vi "Handle Ready State.vi"(0 "reference in":refnum<class "PM_Group.lvclass">, 11 "error in (no error)":errorcluster) -> (4 "reference out":refnum<class "PM_Group.lvclass">, 15 "error out":errorcluster)   [LabVIEW 2019, in "PM_Group.lvclass"]
uses:
  PM_Group.lvclass
  C:/Users/H4001/Documents/GitHub/H4000/src/Device_class/Device.lvclass
  PM_Group.lvclass/PM_Group.ctl
  Device_class/Device.lvclass/Device.ctl
  FPGA/TypeDef/DI index.ctl
  TypeDef/State PMG.ctl
  FPGA_API_class/FPGA API.lvclass
  Device_class/Device.lvclass
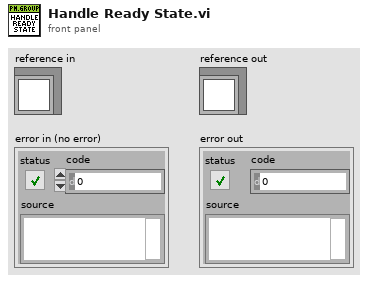
[diagram p1: front panel]
types:
  T1 = typedef "State PMG.ctl" = enum16{"NOT READY", "IDLE", "ACTIVE", "ERROR"}
  T2 = typedef "DI index.ctl" = u8
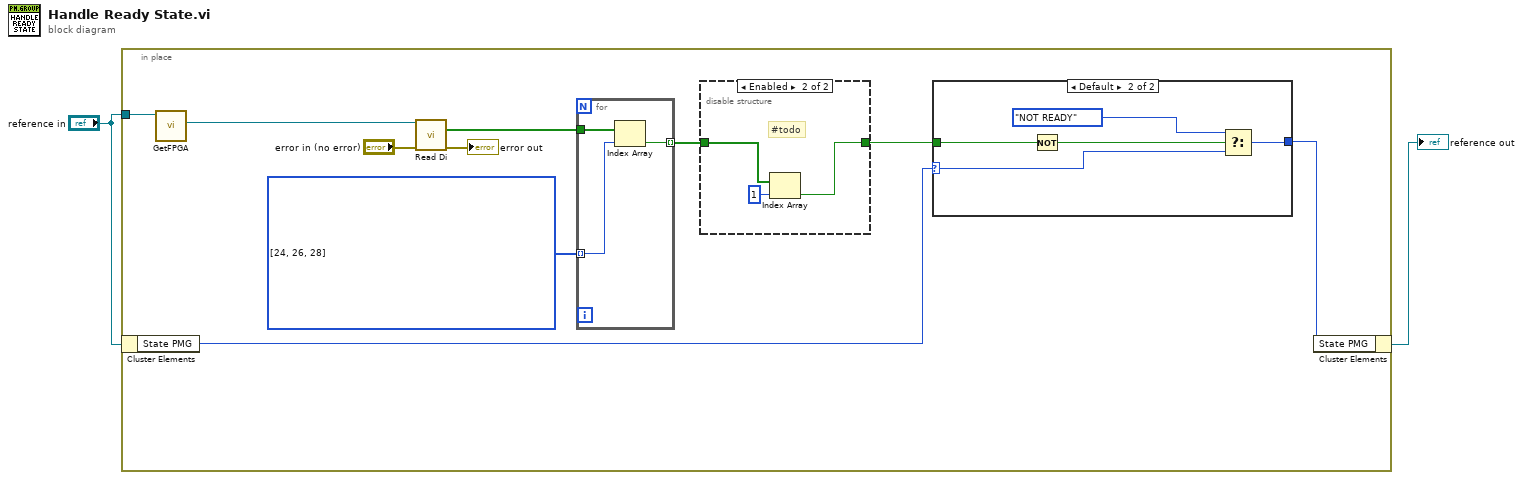
[diagram p0: block diagram]
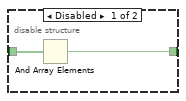
[diagram p2: hidden frame]
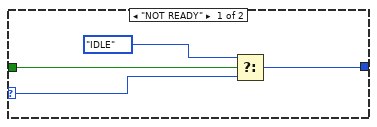
[diagram p3: hidden frame]
diagram:
  n1 = in-place {
    in-place-border: "reference in" -> [w4]
    w11 = T2[] [24, 26, 28] items=["DI 0 [QF1]", "DI 1 [QF2]", "DI 2 [QF3]", "DI 3 [QF4]", "DI 4 [QF5]", "DI 5 [QF6]", "DI 6 [QF7]", "DI 7 [QF8]", "DI 8 [QF9]", "DI 9 [PHASE CONTROL RELAY CONTACTOR [KV1]]", "DI 10 [G1]", "DI 11 [G2]", "DI 12 [RESET BTN [SB1]]", "DI 13 [START BTN [SB2]]", "DI 14 [STOP BTN [SB3]]", "DI 15 [ES BTN [SB4]]", "DI 16 [MANUAL/AUTO MODE SA1]", "DI 17 [[S1]]", "DI 18 [[S2]]", "DI 19 [[S3]]", "DI 20 [[S4]]", "DI 21 [44.1 OPEN]", "DI 22 [44.1 CLOSE]", "DI 23 [CONTACTOR [MK1]]", "DI 24 [AUTOMATIC [QF11]]", "DI 25 [CONTACTOR [MK2]]", "DI 26 [AUTOMATIC [QF12]]", "DI 27 [CONTACTOR [MK3]]", "DI 28 [AUTOMATIC [QF13]]", "DI 29 [44.2 OPEN]", "DI 30 [44.2 CLOSE]"] ("Array")
    n2 = in-place-cluster #1("reference in") -> ("State PMG"=w9:T1)
    n3 = call "GetFPGA.vi"("Device in"=w4) -> ("FPGA API.lvclass"=w3:refnum<class "FPGA API.lvclass">)  [unwired: 10 in]
    n4 = call "Read Di.vi"("FPGA API in"=w3, "error in (no error)"="error in (no error)") -> ("DIs"=w12:bool[], "error out"=→"error out":errorcluster)  [unwired: 11 in, 1 out]
    n5 = for {
      tunnel: w12 -> [w29]
      tunnel: w11 -> [w28] mode=indexing
      tunnel: [w27] -> w10 mode=indexing
      n6 = Index Array(array=w29, index=w28) -> (element=w27:bool)
    }
    n7 = disable-structure shown="Enabled" {
      disable-tunnel: w10 -> [w14 w17]
      disable-tunnel: [w13 w15] -> w8
      frame Disabled {
        n8 = And Array Elements(Boolean array=w14) -> (logical AND=w13:bool)
      }
      frame Enabled {
        # "#todo"
        n9 = Index Array(array=w17, index=1) -> (element=w15:bool)
      }
    }
    n10 = case shown="Default" w9 {
      selector: w9 -> [w20 w25]
      tunnel: w8 -> [w21 w26]
      tunnel: [w18 w23] -> w7
      frame "NOT READY" {
        n11 = Select(t=State_PMG."IDLE", s=w21, f=w20) -> (s? t:f=w18:T1)
      }
      frame Default {
        n12 = Not(x=w26) -> (.not. x?=w22:bool)
        n13 = Select(t=State_PMG."NOT READY", s=w22, f=w25) -> (s? t:f=w23:T1)
      }
    }
    n14 = in-place-cluster #1("State PMG"=w7) -> (→"reference out":refnum<class "PM_Group.lvclass">)
  }
